vi "to string.vi"(8 "error in":errorcluster, 11 "CVT configuration in":refnum<class "testmod configuration.lvclass">) -> (0 "error out":errorcluster, 1 "data":string, 2 "version":string, 3 "CVT configuration out":refnum<class "testmod configuration.lvclass">)   [LabVIEW 2013, in "testmod configuration.lvclass"]
doc: "Provides an interface for saving a module configuration to a file or other serialized data source. It is recommended that all children of this class store data in two sets--data required for its own initialization, and any data required for parent initialization--and that each implementation uses the <b>Call Parent Method</b> primitive to serialize parent information."
uses:
  testmod configuration.lvclass
  <vilib>/NI/Tag Bus Module Framework/module configuration/TBM module configuration.lvclass
  testmod configuration.lvclass/testmod configuration.ctl
  <vilib>/NI/Configuration Framework/serializable configuration/NISE_CEF_serializable configuration.lvclass
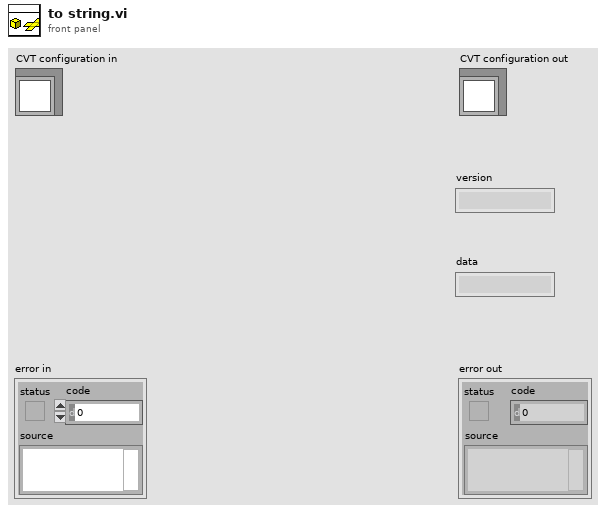
[diagram p1: front panel]
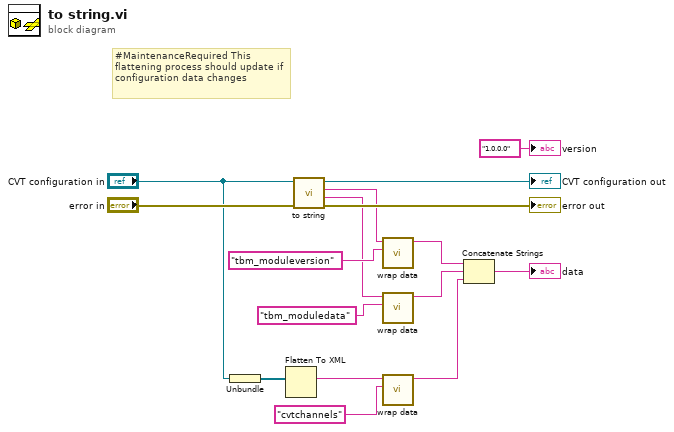
[diagram p0: block diagram]
diagram:
  # "#MaintenanceRequired This flattening process should update if configuration data changes"
  n1 = Unbundle("CVT configuration in") -> (w5:refnum<class "TBM channel.lvclass">[])
  n2 = Flatten To XML(anything=w5) -> (xml string=w4:string)
  n3 = call-parent "to string.vi"("error in"="error in", "module configuration in"="CVT configuration in") -> ("error out"=→"error out":errorcluster, "data"=w8:string, "version"=w9:string, "module configuration out"=→"CVT configuration out":refnum<class "testmod configuration.lvclass">)  [unwired: 6 in]
  n4 = call <vilib>:"wrap data.vi"("identifier"="tbm_moduleversion" ("additional identifier"), "data to wrap"=w9) -> ("wrapped data"=w11:string)  [unwired: 9 in]
  n5 = call <vilib>:"wrap data.vi"("identifier"="tbm_moduledata" ("additional identifier"), "data to wrap"=w8) -> ("wrapped data"=w10:string)  [unwired: 9 in]
  n6 = call <vilib>:"wrap data.vi"("identifier"="cvtchannels" ("additional identifier"), "data to wrap"=w4) -> ("wrapped data"=w3:string)  [unwired: 9 in]
  n7 = Concatenate Strings(w11, w10, w3) -> (→"data":string)
  "version" <- "1.0.0.0" ("version")
